vi "6. VisionFGV.vi"() -> ()   [LabVIEW 2019]
panel:
  in  "Stop Button":bool
  out "Image Start":T1(plugin-control)
  out "Image Grab":T1(plugin-control)
  in  "Grab":bool
  # "c 2022 ReMiSYS All rights reserved."
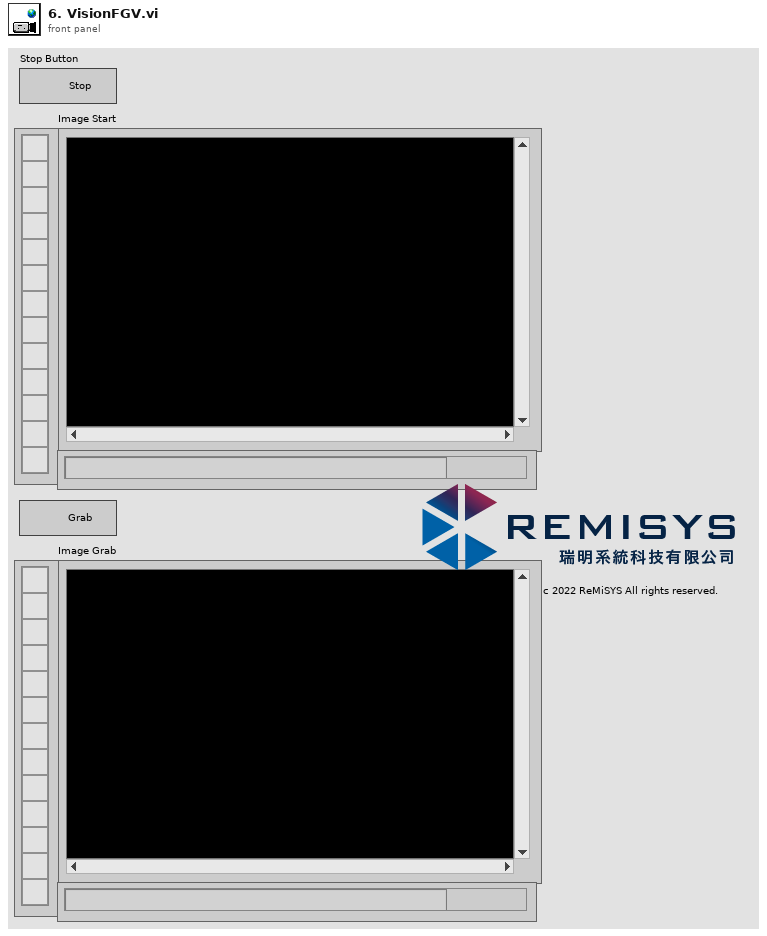
[diagram p1: front panel]
types:
  T1 = typedef "IMAQ Image.ctl" = refnum<image>
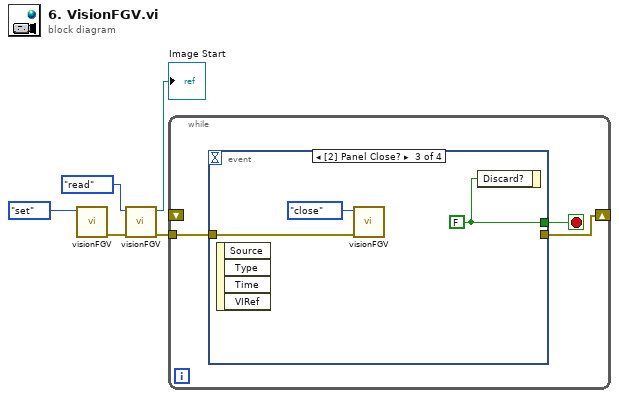
[diagram p0: block diagram]
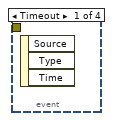
[diagram p2: hidden frame]
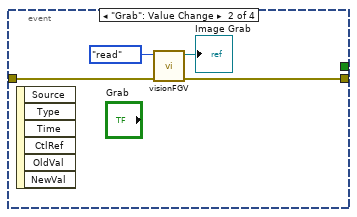
[diagram p3: hidden frame]
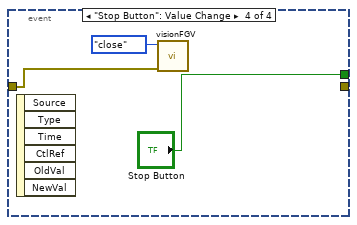
[diagram p4: hidden frame]
diagram:
  n1 = call "visionFGV.vi"("Function"=enum16{"set", "read", "close"}."set") -> ("error out"=w4:errorcluster)  [unwired: 9 in, 1 out]
  n2 = call "visionFGV.vi"("Error In"=w4, "Function"=enum16{"set", "read", "close"}."read") -> ("error out"=w3:errorcluster, "Image Out fgv"=→"Image Start":T1)  [unwired: 8 in]
  n3 = while {
    tunnel: w3 -> [w7]
    shift-right: [w6] -> _
    shift-left: _ -> [_]
    stop <- w8 stop-if-true
    n4 = event shown="[2] Panel Close?" {
      selector: _ -> [_ _ _ _]
      dyn-events: _ -> [_ _ _ _]
      timeout: _ -> [_ _ _ _]
      tunnel: [_ _ w15 "Stop Button"] -> w8
      tunnel: w7 -> [_ w10 w13 w16]
      tunnel: [_ w9 _ _] -> w6
      event Timeout {
        n5 = event-data() -> ()  [unwired: 1 in, 3 out]
      }
      event "Grab": Value Change {
        n6 = event-data() -> ()  [unwired: 1 in, 6 out]
        n7 = call "visionFGV.vi"("Error In"=w10, "Function"=enum16{"set", "read", "close"}."read" ("Function 2")) -> ("error out"=w9:errorcluster, "Image Out fgv"=→"Image Grab":T1)  [unwired: 8 in]
      }
      event Panel Close? {
        w15 = FALSE ("Discard?")
        n8 = event-data() -> ()  [unwired: 1 in, 4 out]
        n9 = call "visionFGV.vi"("Error In"=w13, "Function"=enum16{"set", "read", "close"}."close") -> ()  [unwired: 8 in, 2 out]
        n10 = event-data("Discard?"=w15) -> ()  [unwired: 1 in, 1 out]
      }
      event "Stop Button": Value Change {
        n11 = event-data() -> ()  [unwired: 1 in, 6 out]
        n12 = call "visionFGV.vi"("Error In"=w16, "Function"=enum16{"set", "read", "close"}."close") -> ()  [unwired: 8 in, 2 out]
      }
    }
  }
